vi "Get Hwnd and Hide.vi"(0 "Doc Name":string, 5 "Shell Name":string, 11 "error in (no error)":errorcluster) -> (4 "hwnd":u32, 6 "Shell hwnd":u32, 15 "error out":errorcluster)   [LabVIEW 2016, in "Document.lvclass"]
uses:
  Document.lvclass
  Child Classes/Py Doc/Py Doc.lvclass
  user32.dll
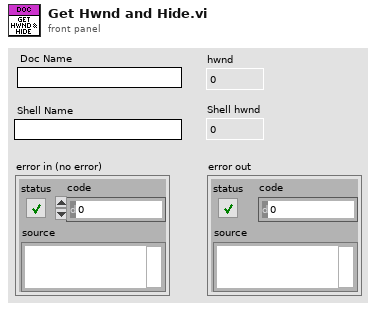
[diagram p1: front panel]
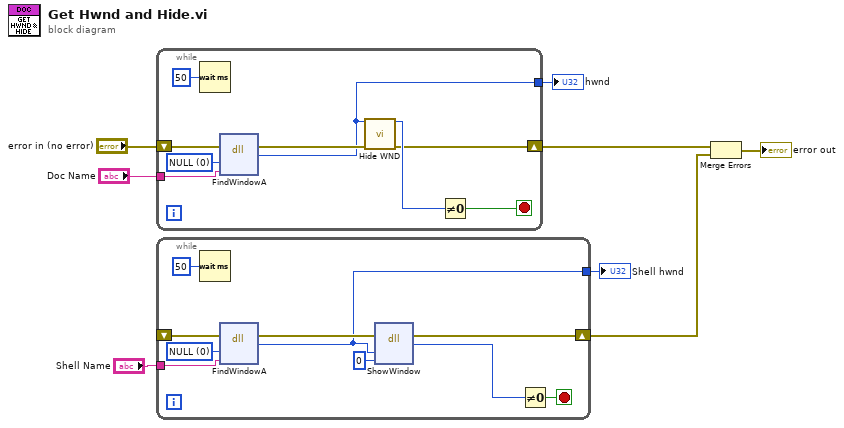
[diagram p0: block diagram]
diagram:
  n1 = while {
    tunnel: "Doc Name" -> [w14]
    tunnel: [w11] -> w8
    shift-right: [w10] -> w4
    shift-left: "error in (no error)" -> [w15]
    stop <- w9 stop-if-true
    w17 = 0 items=["NULL"]
    n2 = Wait (ms)(milliseconds to wait=u32 50) -> ()  [unwired: 1 out]
    n3 = dll-call lib="user32.dll" fn="FindWindowA"(error in=w15, "lpzsClassName"=w17, "lpzsWindowName"=w14) -> (error out=w16:errorcluster, "hwnd"=w11:u32)  [unwired: 4 in, 1 out]
    n4 = call "Hide WND.vi"("hwnd"=w11, "error in (no error)"=w16) -> ("bool"=w12:u32, "error out"=w10:errorcluster)  [unwired: 12 in]
    n5 = Not Equal To 0?(x=w12) -> (x != 0?=w9:bool)
  }
  "hwnd" <- w8
  n6 = while {
    tunnel: "Shell Name" -> [w24]
    tunnel: [w22] -> w1
    shift-right: [w19] -> w3
    shift-left: _ -> [w25]
    stop <- w21 stop-if-true
    w27 = 0 items=["NULL"]
    n7 = Wait (ms)(milliseconds to wait=u32 50) -> ()  [unwired: 1 out]
    n8 = dll-call lib="user32.dll" fn="FindWindowA"(error in=w25, "lpzsClassName"=w27, "lpzsWindowName"=w24) -> (error out=w26:errorcluster, "hwnd"=w22:u32)  [unwired: 4 in, 1 out]
    n9 = dll-call lib="user32.dll" fn="ShowWindow"(error in=w26, "hwnd"=w22, "nCmdShow"=u32 0) -> (error out=w19:errorcluster, "bool"=w18:u32)  [unwired: 4 in, 1 out]
    n10 = Not Equal To 0?(x=w18) -> (x != 0?=w21:bool)
  }
  "Shell hwnd" <- w1
  n11 = Merge Errors(w4, w3) -> (→"error out":errorcluster)
